vi "TTL.vi"(0 "error in":errorcluster, 5 "Amount of Points":i32, 7 "Duty Cycle":dbl=0.01 min=0.01 max=0.99) -> (4 "error out":errorcluster, 6 "TTL wave array":dbl[](array[numeric]))   [LabVIEW 2020]
panel:
  out "Waveform Graph":dbl[](graph)
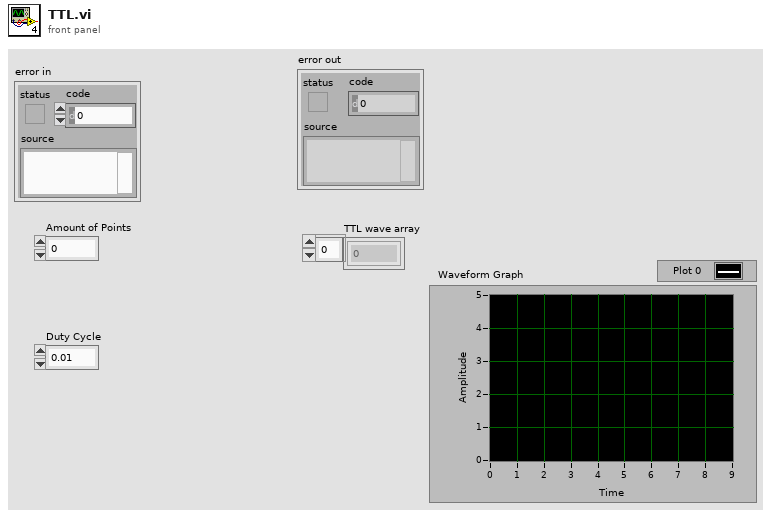
[diagram p1: front panel]
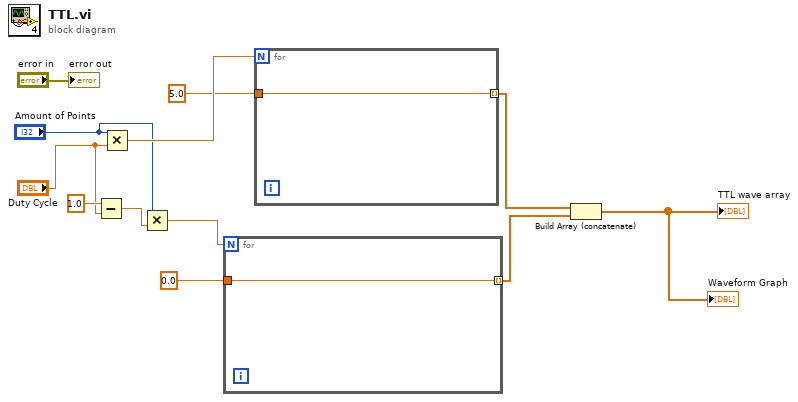
[diagram p0: block diagram]
diagram:
  n1 = Subtract(x=1.0, y="Duty Cycle") -> (x-y=w6:dbl)
  n2 = Multiply(x="Amount of Points", y="Duty Cycle") -> (x*y=w11:dbl)
  n3 = Multiply(x="Amount of Points", y=w6) -> (x*y=w4:dbl)
  n4 = for {
    N: w4 -> [_]
    tunnel: 0.0 -> [w13]
    tunnel: [w13] -> w2 mode=indexing
  }
  n5 = for {
    N: w11 -> [_]
    tunnel: 5.0 -> [w14]
    tunnel: [w14] -> w3 mode=indexing
  }
  n6 = Build Array (concatenate)(w3, w2) -> (→"TTL wave array" →"Waveform Graph":dbl[])
  "error out" <- "error in"
